vi "Hide.vi"(8 "error in (no error)":errorcluster, 11 "loop data in":T1) -> (0 "error out":errorcluster, 3 "loop data out":T1)   [LabVIEW 2021, in "TipStripOOPanel.lvlib"]
uses:
  TipStripOOPanel.lvlib
  Loop Data Parent.ctl
  <vilib>/IlluminatedG/IG OOPanel/OOPanel/Manager/Manager.lvclass
  Classes/TipPanel/TipPanel.lvclass
  PanelMap.ctl
  PanelMapData.ctl
  Classes/TipPanel/ToPanelUEWrapper.ctl
  Classes/TipPanel/ToPanelUE.ctl
  <vilib>/Futures/Futures/Promise/Promise.lvclass
  refs.ctl
  <vilib>/Utility/miscctls.llb/LVRectTypeDef.ctl
  <vilib>/Utility/miscctls.llb/LVBoundsTypeDef.ctl
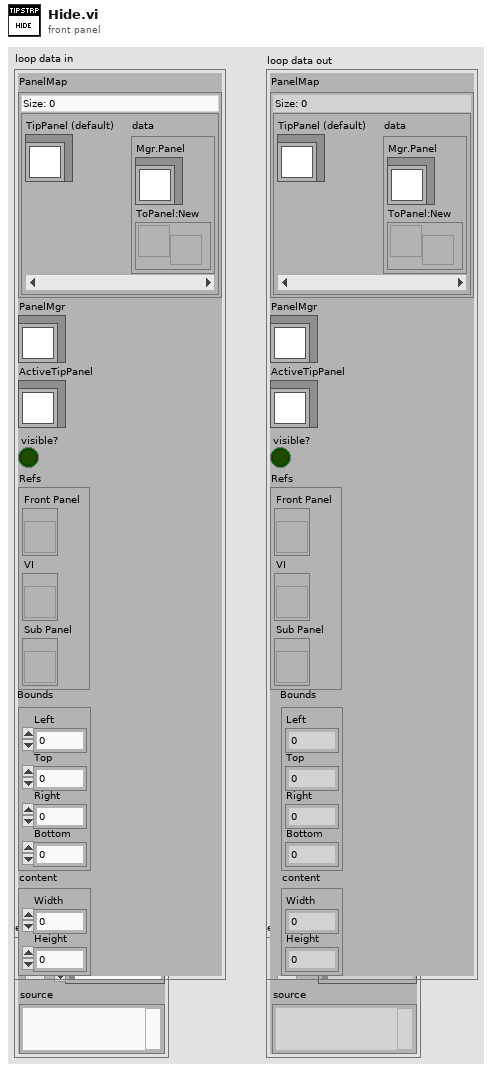
[diagram p1: front panel]
types:
  T1 = typedef "TipStripOOPanel.lvlib/Loop Data Parent.ctl" = cluster{"PanelMap":T2, "PanelMgr":refnum<class "Manager.lvclass">, "ActiveTipPanel":refnum<class "TipPanel.lvclass">, "visible?":bool, "Refs":T4, "Bounds":T5, "content":T6}
  T2 = typedef "TipStripOOPanel.lvlib/PanelMap.ctl" = map{refnum<class "TipPanel.lvclass">, T3}
  T3 = typedef "TipStripOOPanel.lvlib/PanelMapData.ctl" = cluster{"Mgr.Panel":refnum<class "TipPanel.lvclass">, "ToPanel:New":refnum<user-event>}
  T4 = typedef "TipStripOOPanel.lvlib/refs.ctl" = cluster{"Front Panel":refnum<vi>, "VI":refnum<vi>, "Sub Panel":refnum<vi>}
  T5 = typedef "LVRectTypeDef.ctl" = cluster{"Left":i16, "Top":i16, "Right":i16, "Bottom":i16}
  T6 = typedef "LVBoundsTypeDef.ctl" = cluster{"Width":u32, "Height":u32}
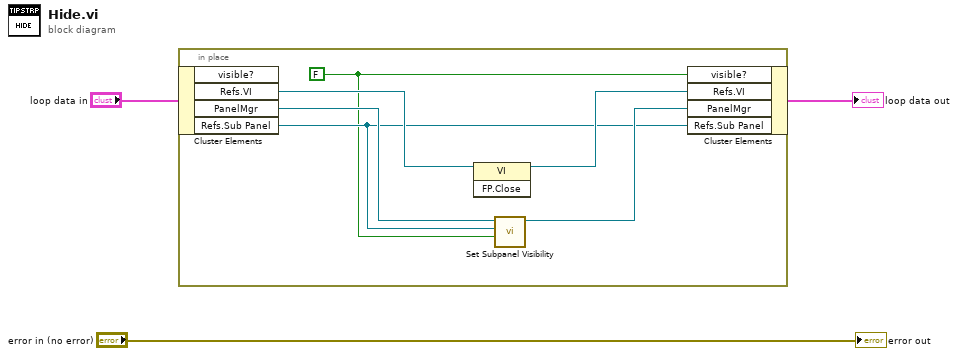
[diagram p0: block diagram]
diagram:
  n1 = in-place {
    w4 = FALSE ("visible?")
    n2 = in-place-cluster #1("loop data in") -> ("Refs.VI"=w9:refnum<vi>, "PanelMgr"=w7:refnum<class "Manager.lvclass">, "Refs.Sub Panel"=w5:refnum<vi>)  [unwired: 1 out]
    n3 = invoke class="VI" method="FP.Close"(reference=w9) -> (reference out=w8:refnum<vi>)  [unwired: 2 in, 2 out]
    n4 = call <vilib>:"Set Subpanel Visibility.vi"("Visible"=w4, "SubPanel"=w5, "Manager in"=w7) -> ("Manager out"=w6:refnum<class "Manager.lvclass">)  [unwired: 7 in, 1 out]
    n5 = in-place-cluster #1("visible?"=w4, "Refs.VI"=w8, "PanelMgr"=w6, "Refs.Sub Panel"=w5) -> (→"loop data out":T1)
  }
  "error out" <- "error in (no error)"
